vi "Insert Into Map.vi"(0 "DBMap in":refnum<class "DBMap.lvclass">, 5 "Key":string, 7 "File Data":T1, 11 "error in (no error)":errorcluster {"code" format="Error %.0f"}) -> (4 "DBMap out":refnum<class "DBMap.lvclass">, 15 "error out":errorcluster {"code" format="Error %.0f"})   [LabVIEW 2024, in "DBMap.lvclass"]
uses:
  DBMap.lvclass
  DBMap.lvclass/DBMap.ctl
  <vilib>/drjdpowell/SQLite Library/SQL Statement/SQL Statement.lvclass/SQL Statement.ctl
  <vilib>/drjdpowell/SQLite Library/SQL Connection/Connection.lvclass
  <vilib>/drjdpowell/SQLite Library/SQL Statement/SQL Statement.lvclass
  File Metadata.ctl
  Node.ctl
  Source to Sink Array.ctl
  File Data.ctl
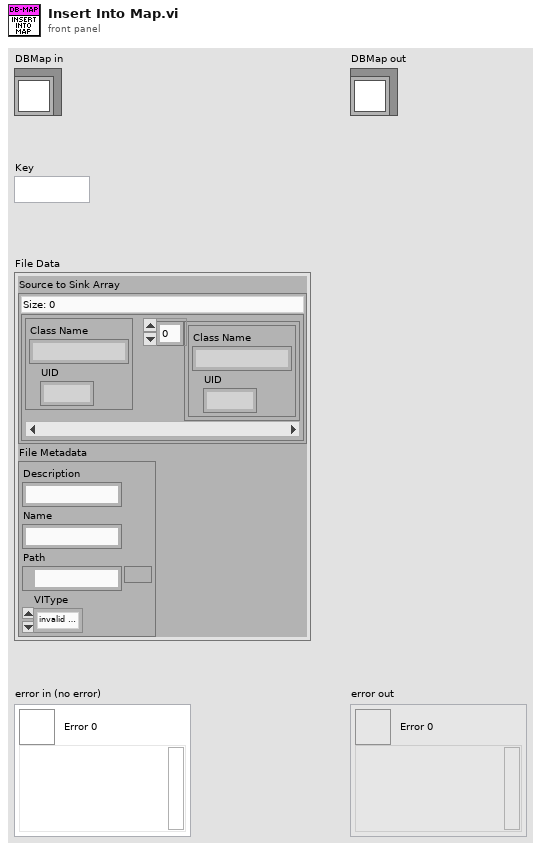
[diagram p1: front panel]
types:
  T1 = typedef "File Data.ctl" = cluster{"Source to Sink Array":T2, "File Metadata":T4}
  T2 = typedef "Source to Sink Array.ctl" = map{T3, T3[]}
  T3 = typedef "Node.ctl" = cluster{"Class Name":string, "UID":i32}
  T4 = typedef "File Metadata.ctl" = cluster{"Description":string, "Name":string, "Path":path, "VIType":enum32{"invalid VI type", "Standard VI", "Control VI", "Global VI", "Polymorphic VI", "Configuration VI", "SubSystem", "Facade VI", "Method VI", "Statechart Diagram VI"}}
  T5 = typedef "Semaphore RefNum" = refnum<k1>
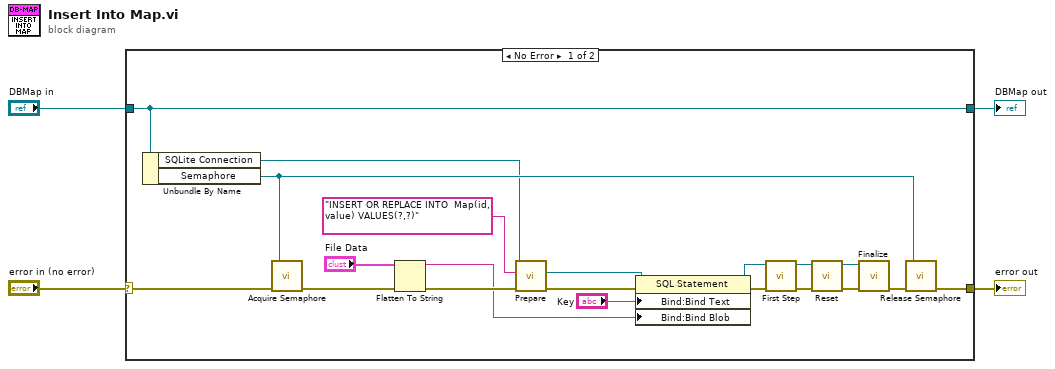
[diagram p0: block diagram]
diagram:
  n1 = case shown="No Error" "error in (no error)" {
    selector: "error in (no error)" -> [w23 w26]
    tunnel: [w22 w26] -> w3
    tunnel: [w24 w25] -> w1
    tunnel: "DBMap in" -> [w24 w25]
    frame No Error {
      n2 = Unbundle By Name(w24) -> ("SQLite Connection"=w6:refnum<class "Connection.lvclass">, "Semaphore"=w21:T5)
      n3 = call <vilib>:"Acquire Semaphore.vi"("error in (no error)"=w23, "semaphore"=w21) -> ("error out"=w8:errorcluster)  [unwired: 3 in, 2 out]
      n4 = Flatten To String(anything="File Data", error in (no error)=w8) -> (data string=w11:string, error out=w20:errorcluster)  [unwired: 2 in, 1 out]
      n5 = call <vilib>:"Prepare.vi"("error in (no error)"=w20, "SQL"="INSERT OR REPLACE INTO  Map(id, value) VALUES(?,?)", "SQLite Connection in"=w6) -> ("error out"=w14:errorcluster, "SQL Statement"=w13:refnum<class "SQL Statement.lvclass">)  [unwired: 4 in, 3 out]
      n6 = property class="SQL Statement"(reference=w13, error in=w14, "Bind:Bind Text"="Key", "Bind:Bind Blob"=w11) -> (reference out=w17:refnum<class "SQL Statement.lvclass">, error out=w18:errorcluster)
      n7 = call <vilib>:"First Step.vi"("error in (no error)"=w18, "SQL Statement in"=w17) -> ("error out"=w16:errorcluster, "SQL Statement"=w15:refnum<class "SQL Statement.lvclass">)  [unwired: 7 in, 1 out]
      n8 = call <vilib>:"Reset.vi"("error in (no error)"=w16, "SQL Statement in"=w15) -> ("error out"=w10:errorcluster, "SQL Statement"=w9:refnum<class "SQL Statement.lvclass">)  [unwired: 8 in]
      n9 = call <vilib>:"Finalize.vi"("error in (no error)"=w10, "SQL Statement in"=w9) -> ("error out"=w7:errorcluster)  [unwired: 9 in]
      n10 = call <vilib>:"Release Semaphore.vi"("error in (no error)"=w7, "semaphore"=w21) -> ("error out"=w22:errorcluster)  [unwired: 4 in, 1 out]
    }
    frame Error {
    }
  }
  "error out" <- w3
  "DBMap out" <- w1
